vi "Set Quality of Run Observalbes.vi"(8 "error in (no error)":errorcluster, 10 "Obsv to check":T1(array[cluster]), 11 "Schedule Cell in":refnum<class "Schedule Cell.lvclass">) -> (0 "error out":errorcluster, 3 "Schedule Cell out":refnum<class "Schedule Cell.lvclass">)   [LabVIEW 2020, in "CIRCUS_uServices.lvlib" / "Run Utilities.lvlib" / "Schedule Cell.lvclass"]
uses:
  Schedule Cell.lvclass
  Run Instance/Run Instance.lvclass
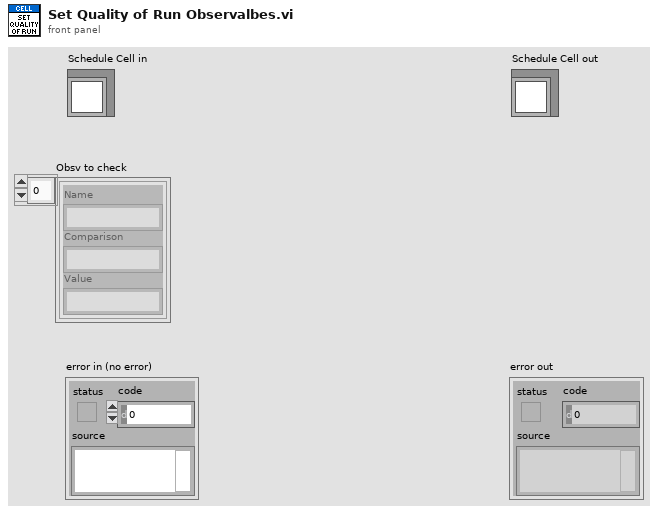
[diagram p1: front panel]
types:
  T1 = cluster{"Name":string, "Comparison":string, "Value":string}[]
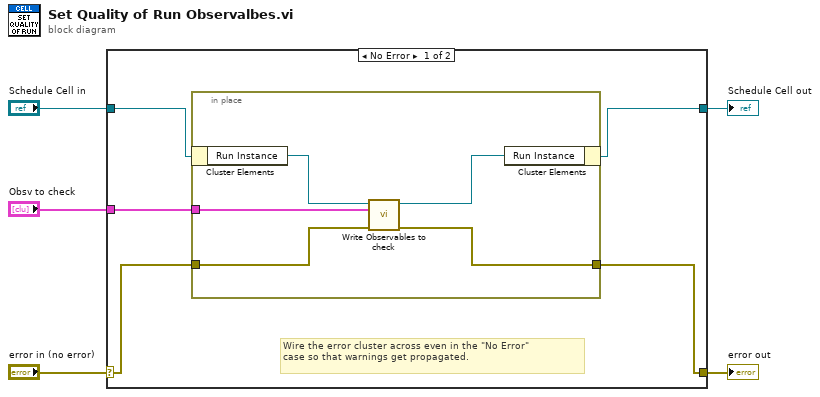
[diagram p0: block diagram]
diagram:
  n1 = case shown="No Error" "error in (no error)" {
    selector: "error in (no error)" -> [w8 w17]
    tunnel: [w7 w17] -> w4
    tunnel: [w9 w16] -> w2
    tunnel: "Schedule Cell in" -> [w10 w16]
    tunnel: "Obsv to check" -> [w6 _]
    frame No Error {
      # "Wire the error cluster across even in the \"No Error\"\ncase so that warnings get propagated."
      n2 = in-place {
        in-place-border: w8 -> [w13]
        in-place-border: [w12] -> w7
        in-place-border: w6 -> [w11]
        n3 = in-place-cluster #1(w10) -> ("Run Instance"=w15:refnum<class "Run Instance.lvclass">)
        n4 = call-dynamic "Write Observables to check.vi"("error in (no error)"=w13, "Obsv to check"=w11, "Run Instance in"=w15) -> ("error out"=w12:errorcluster, "Run Instance out"=w14:refnum<class "Run Instance.lvclass">)  [unwired: 7 in]
        n5 = in-place-cluster #1("Run Instance"=w14) -> (w9:refnum<class "Schedule Cell.lvclass">)
      }
    }
    frame Error {
    }
  }
  "error out" <- w4
  "Schedule Cell out" <- w2
